vi "Poly_fit.vi"(0 "Input Y array":dbl[](array[numeric]) format="%.4f", 2 "Input X array":dbl[](array[numeric]) format="%.3f", 4 "polynomial order":i32=2, 5 "Point selector":cluster{"Y":dbl, "X":dbl, "switch":bool}[](array[cluster]) {"X" format="%.2f"; "Y" format="%.2f"}) -> (1 "Coefficients":dbl[](array[numeric]) format="%.2f", 6 "Calib const":string[][](array[string]), 7 "Calibration plot":cluster{cluster{dbl, dbl}[]}[](graph), 8 "Point selector":cluster{"Y":dbl, "X":dbl, "switch":bool}[](array[cluster]) {"X" format="%.2f"; "Y" format="%.2f"})   [LabVIEW 2013]
uses:
  <vilib>/Analysis/baseanly.llb/Mean (DBL).vi
  <vilib>/Analysis/NI_AALPro.lvlib
  <vilib>/Analysis/NI_AALBase.lvlib
panel:
  in  "Type":cluster{"Y":dbl, "X":dbl, "switch":bool}={"Y"=10.144154930121, "X"=9.20412, "switch"=FALSE} {"X" format="%.2f"; "Y" format="%.2f"}
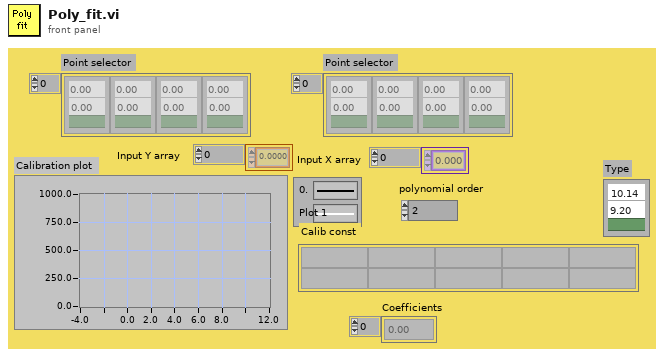
[diagram p1: front panel]
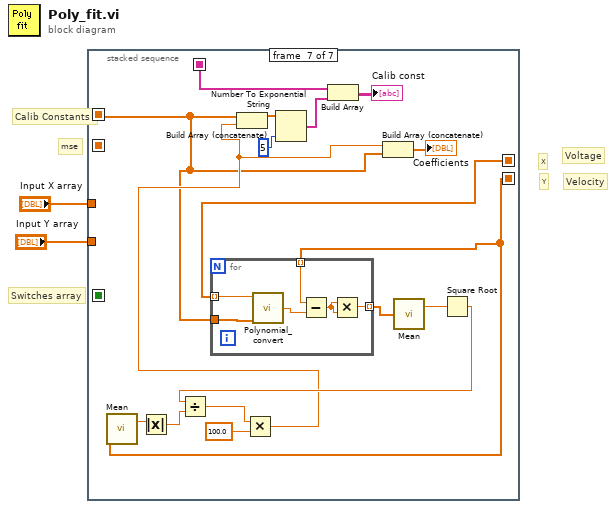
[diagram p0: block diagram]
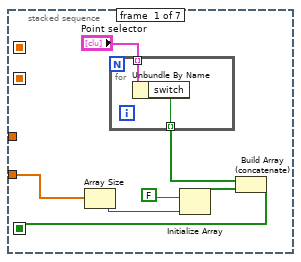
[diagram p2: hidden frame]
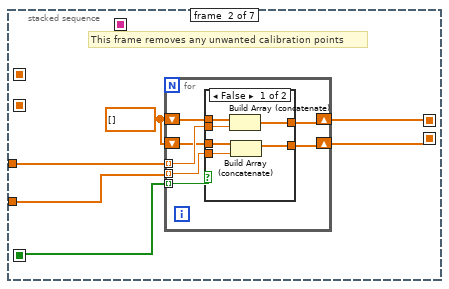
[diagram p3: hidden frame]
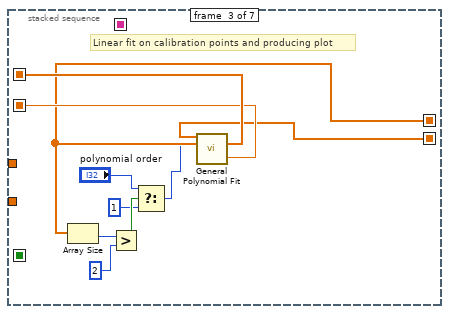
[diagram p5: hidden frame]
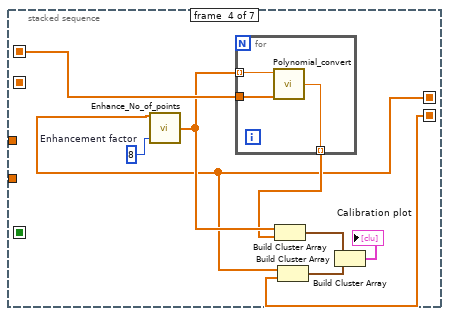
[diagram p6: hidden frame]
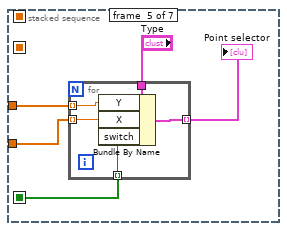
[diagram p7: hidden frame]
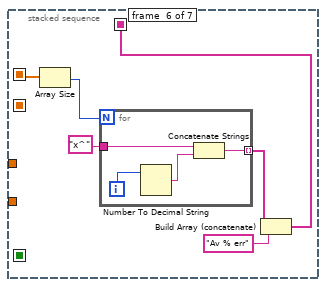
[diagram p8: hidden frame]
diagram:
  # "mse"
  # "Calib Constants"
  # "Voltage"
  # "Velocity"
  # "Switches array"
  # "X"
  # "Y"
  n1 = stacked-sequence {
    seq-local: [_ w17 _ _ _ _ _] -> [_ _ w35 w44 _ _ w76]
    seq-local: [_ w16 _ _ _ _ _] -> [_ _ w40 w43 _ _ w78]
    seq-local: [w7 _ _ _ _ _ _] -> [_ w13 _ _ w56 _ _]
    seq-local: [_ _ w42 _ _ _ _] -> [_ _ _ w47 _ w68 w75]
    seq-local: [_ _ w41 _ _ _ _] -> [_ _ _ _ _ _ _]
    seq-local: [_ _ _ _ _ w65 _] -> [_ _ _ _ _ _ w88]
    tunnel: "Input Y array" -> [w3 w14 _ _ w57 _ _]
    tunnel: "Input X array" -> [_ w15 _ _ w58 _ _]
    frame #0 {
      n2 = Array Size(array=w3) -> (size(s)=w5:i32)
      n3 = for {
        tunnel: "Point selector" -> [w11] mode=indexing
        tunnel: [w10] -> w8 mode=indexing
        n4 = Unbundle By Name(w11) -> ("switch"=w10:bool)
      }
      n5 = Initialize Array(FALSE, w5) -> (w4:bool[])
      n6 = Build Array (concatenate)(w8, w4) -> (w7:bool[])
    }
    frame #1 {
      w12 = dbl[] []
      # "This frame removes any unwanted calibration points"
      n7 = for {
        shift-right: [w18] -> w16
        shift-left: w12 -> [w20]
        shift-right: [w19] -> w17
        shift-left: w12 -> [w21]
        tunnel: w13 -> [w22] mode=indexing
        tunnel: w14 -> [w23] mode=indexing
        tunnel: w15 -> [w24] mode=indexing
        n8 = case shown="False" w22 {
          tunnel: [w25 w31] -> w18
          tunnel: [w26 w32] -> w19
          tunnel: w20 -> [w27 w31]
          tunnel: w21 -> [w28 w32]
          tunnel: w23 -> [w29 _]
          tunnel: w24 -> [w30 _]
          frame False {
            n9 = Build Array (concatenate)(w28, w30) -> (w26:dbl[])
            n10 = Build Array (concatenate)(w27, w29) -> (w25:dbl[])
          }
          frame True {
          }
        }
      }
    }
    frame #2 {
      # "Linear fit on calibration points and producing plot"
      n11 = Array Size(array=w35) -> (size(s)=w39:i32)
      n12 = Greater?(x=w39, y=2) -> (0:w36:bool)
      n13 = Select(t="polynomial order", s=w36, f=1) -> (s? t:f=w33:i32)
      n14 = call <vilib>:"General Polynomial Fit.vi"("Y"=w40, "polynomial order"=w33, "X"=w35) -> ("Polynomial Coefficients"=w42:dbl[], "residue"=w41:dbl)  [unwired: 9 in, 2 out]
    }
    frame #3 {
      w48 = 8  # Enhancement factor
      n15 = call "Enhance_No_of_points.vi"("Enhancement factor"=w48, "Input"=w44) -> ("Output"=w46:dbl[])  [unwired: 3 out]
      n16 = for {
        tunnel: w47 -> [w54]
        tunnel: w46 -> [w53] mode=indexing
        tunnel: [w52] -> w45 mode=indexing
        n17 = call "Polynomial_convert.vi"("Calib constants"=w54, "Voltage"=w53) -> ("Eng Values"=w52:dbl)  [unwired: 4 out]
      }
      n18 = Build Cluster Array(w46, w45) -> (w51:cluster{dbl, "Eng Values":dbl}[])
      n19 = Build Cluster Array(w44, w43) -> (w50:cluster{dbl, dbl}[])
      n20 = Build Cluster Array(w51, w50) -> (→"Calibration plot":cluster{cluster{dbl, "Eng Values":dbl}[]}[])
    }
    frame #4 {
      n21 = for {
        tunnel: "Type" -> [w64]
        tunnel: w58 -> [w63] mode=indexing
        tunnel: w57 -> [w62] mode=indexing
        tunnel: w56 -> [w61] mode=indexing
        tunnel: [w60] -> w55 mode=indexing
        n22 = Bundle By Name(cluster=w64, "Y"=w63, "X"=w62, "switch"=w61) -> (w60:cluster{"Y":dbl, "X":dbl, "switch":bool})
      }
      "Point selector" <- w55
    }
    frame #5 {
      n23 = Array Size(array=w68) -> (size(s)=w67:i32)
      n24 = for {
        N: w67 -> [_]
        tunnel: "x^" -> [w72]
        tunnel: [w71] -> w66 mode=indexing
        i -> [w74]
        n25 = Number To Decimal String(number=w74) -> (decimal integer string=w73:string)  [unwired: 1 out]
        n26 = Concatenate Strings(w72, w73) -> (w71:string)
      }
      n27 = Build Array (concatenate)(w66, "Av % err") -> (w65:string[])
    }
    frame #6 {
      n28 = call-poly <vilib>:"Mean.vi"("X"=w78) -> ("mean"=w85:dbl)  [unwired: 1 out]
      n29 = Absolute Value(x=w85) -> (abs(x)=w82:dbl)
      n30 = for {
        tunnel: w75 -> [w97]
        tunnel: w76 -> [w96] mode=indexing
        tunnel: w78 -> [w94] mode=indexing
        tunnel: [w92] -> w80 mode=indexing
        n31 = call "Polynomial_convert.vi"("Calib constants"=w97, "Voltage"=w96) -> ("Eng Values"=w95:dbl)  [unwired: 4 out]
        n32 = Subtract(x=w94, y=w95) -> (x-y=w93:dbl)
        n33 = Multiply(x=w93, y=w93) -> (x*y=w92:dbl)
      }
      n34 = call-poly <vilib>:"Mean.vi"("X"=w80) -> ("mean"=w79:dbl)  [unwired: 1 out]
      n35 = Square Root(x=w79) -> (sqrt(x)=w83:dbl)
      n36 = Divide(x=w83, y=w82) -> (x/y=w81:dbl)
      n37 = Multiply(x=w81, y=100.0) -> (x*y=w77:dbl)
      n38 = Build Array (concatenate)(w75, w77) -> (w91:dbl[])
      n39 = Number To Exponential String(number=w91, precision (6)=i16 5) -> (E-format string=w90:string[])  [unwired: 2 out]
      n40 = Build Array(w88, w90) -> (→"Calib const":string[][])
      n41 = Build Array (concatenate)(w77, w75) -> (→"Coefficients":dbl[])
    }
  }
